vi "Check for spark.vi"(8 "Threshold (uA)":dbl, 11 "Currents (uA)":dbl[](array[numeric])) -> (3 "Spark?":bool)   [LabVIEW 2018]
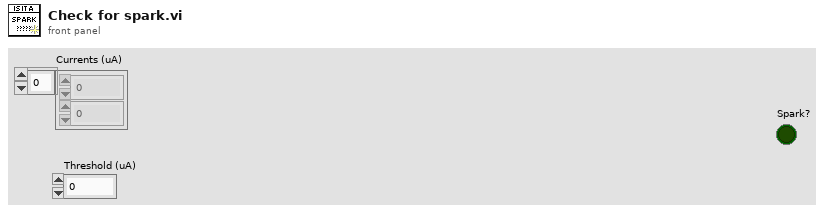
[diagram p1: front panel]
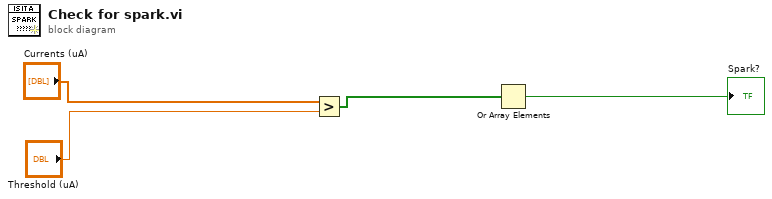
[diagram p0: block diagram]
diagram:
  n1 = Greater?(x="Currents (uA)", y="Threshold (uA)") -> (0:w2:bool[])
  n2 = Or Array Elements(Boolean array=w2) -> (logical OR=→"Spark?":bool)
